vi "AdvanceTable_initRef.vi"(0 "AdvanceTable in":refnum<class "AdvanceTable.lvclass">, 5 "AdvanceTable":refnum<vi>, 7 "ItemsArray":refnum<vi>[](array[refnum]), 9 "RefOfScroll":refnum<vi>, 11 "error in (no error)":errorcluster) -> (4 "AdvanceTable out":refnum<class "AdvanceTable.lvclass">, 15 "error out":errorcluster)   [LabVIEW 2015, in "ActorManagement.lvlib" / "AdvanceTable.lvclass"]
uses:
  AdvanceTable.lvclass
  AdvanceTable.lvclass/AdvanceTable.ctl
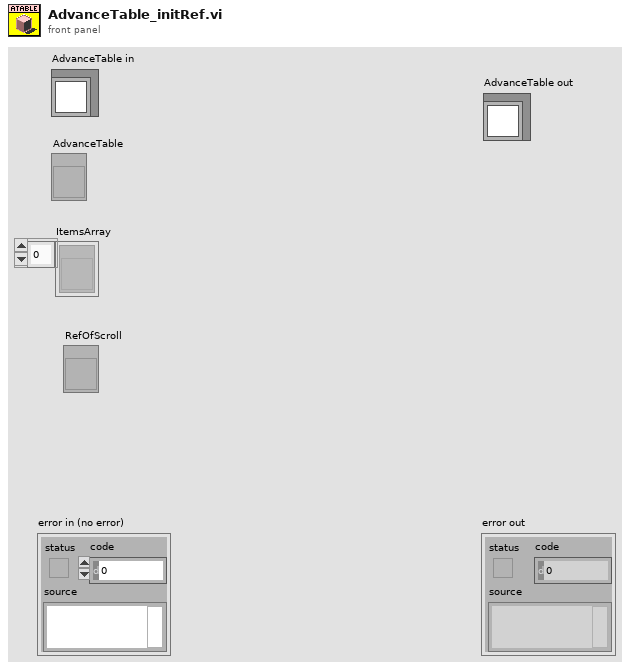
[diagram p1: front panel]
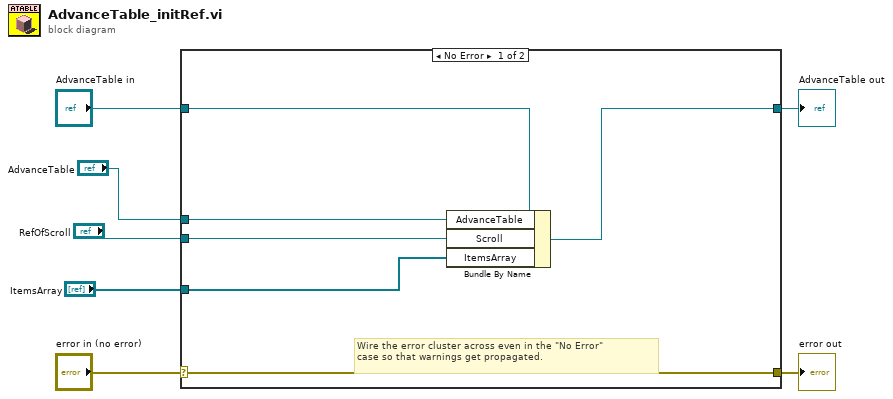
[diagram p0: block diagram]
diagram:
  n1 = case shown="No Error" "error in (no error)" {
    selector: "error in (no error)" -> [w13 w15]
    tunnel: [w13 w15] -> w6
    tunnel: [w11 w14] -> w4
    tunnel: "AdvanceTable in" -> [w12 w14]
    tunnel: "RefOfScroll" -> [w10 _]
    tunnel: "ItemsArray" -> [w9 _]
    tunnel: "AdvanceTable" -> [w8 _]
    frame No Error {
      # "Wire the error cluster across even in the \"No Error\"\ncase so that warnings get propagated."
      n2 = Bundle By Name(cluster=w12, "AdvanceTable"=w8, "Scroll"=w10, "ItemsArray"=w9) -> (w11:refnum<class "AdvanceTable.lvclass">)
    }
    frame Error {
    }
  }
  "error out" <- w6
  "AdvanceTable out" <- w4
